vi "FT10_M4X Configure Horizontal.vi"(0 "Card Handle in":u32, 5 "memsize":i32=16384, 7 "posttrigger (samples)":i32=8192, 9 "sample rate (Hz)":i32=130000000, 11 "error in (no error)":errorcluster) -> (4 "Card Handle out":u32, 15 "error out":errorcluster)   [LabVIEW 2015]
doc: "Copy of \"M4X_Configure Horizontal.vi\" from HWT_Lillis_7854.lvproj"
uses:
  spcm_win32.dll
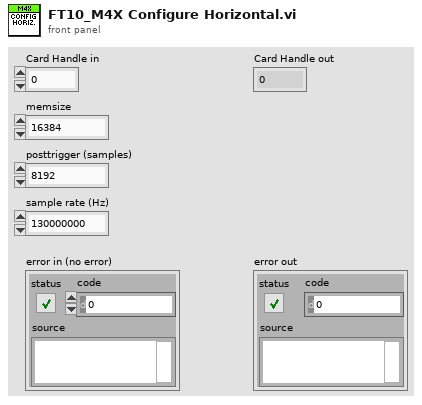
[diagram p1: front panel]
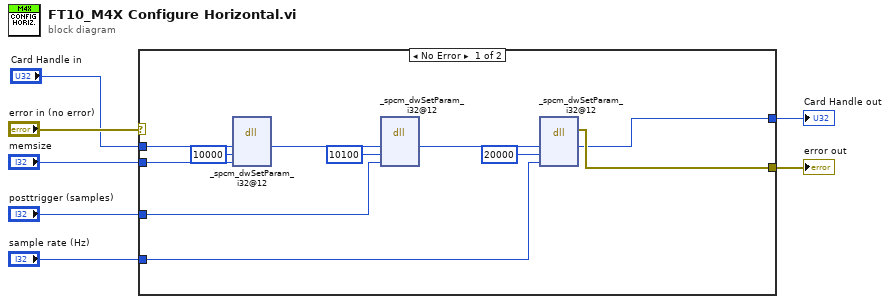
[diagram p0: block diagram]
diagram:
  n1 = case shown="No Error" "error in (no error)" {
    selector: "error in (no error)" -> [_ w20]
    tunnel: "Card Handle in" -> [w18 w19]
    tunnel: "posttrigger (samples)" -> [w13 _]
    tunnel: "memsize" -> [w16 _]
    tunnel: [w9 w20] -> w4
    tunnel: [w8 w19] -> w5
    tunnel: "sample rate (Hz)" -> [w10 _]
    frame No Error {
      n2 = dll-call lib="spcm_win32.dll" fn="_spcm_dwSetParam_i32@12" label="Set Memsize"("hDrv"=w18, "lRegister"=10000 ("Reg"), "lValue"=w16) -> ("hDrv"=w14:u32)  [unwired: 6 in, 2 out]
      n3 = dll-call lib="spcm_win32.dll" fn="_spcm_dwSetParam_i32@12" label="Set PostTrigger"("hDrv"=w14, "lRegister"=10100 ("Reg"), "lValue"=w13) -> ("hDrv"=w12:u32)  [unwired: 6 in, 2 out]
      n4 = dll-call lib="spcm_win32.dll" fn="_spcm_dwSetParam_i32@12" label="Set SampleRate"("hDrv"=w12, "lRegister"=20000 ("Reg"), "lValue"=w10) -> (error out=w9:errorcluster, "hDrv"=w8:u32)  [unwired: 6 in, 1 out]
    }
    frame Error {
    }
  }
  "Card Handle out" <- w5
  "error out" <- w4
